vi "VILab.vi"() -> ()   [LabVIEW 2026, in "VILab.lvlib"]
uses:
  VILab.lvlib
  CTLs/VILab State Data.ctl
  Classes/Tree Manager/Tree Manager.lvclass
  CTLs/Resource.ctl
  Classes/Data Item/Data Item.lvclass
  <vilib>/Utility/error.llb/Clear Errors.vi
  SubVIs/Decompose VI (Refnum).vi
  SubVIs/FaKI State Machine/FaKI State Machine.lvlib
panel:
  in  "Dissect":bool
  in  "Rebuild":bool
  in  "Properties":bool
  in  "Clone":bool
  in  "Delete":bool
  in  "Add":bool
  in  "Tree":string(tree)
  # "WARNING:\nThis unofficial utility has NO WARRANTY and uses internal LabVIEW functionality that is NOT supported by National Instruments.\nYou will very likely crash LabVIEW and create insane/corrupted VI's, so use this at your own risk. But that's all part of the Fun™, right? ;)"
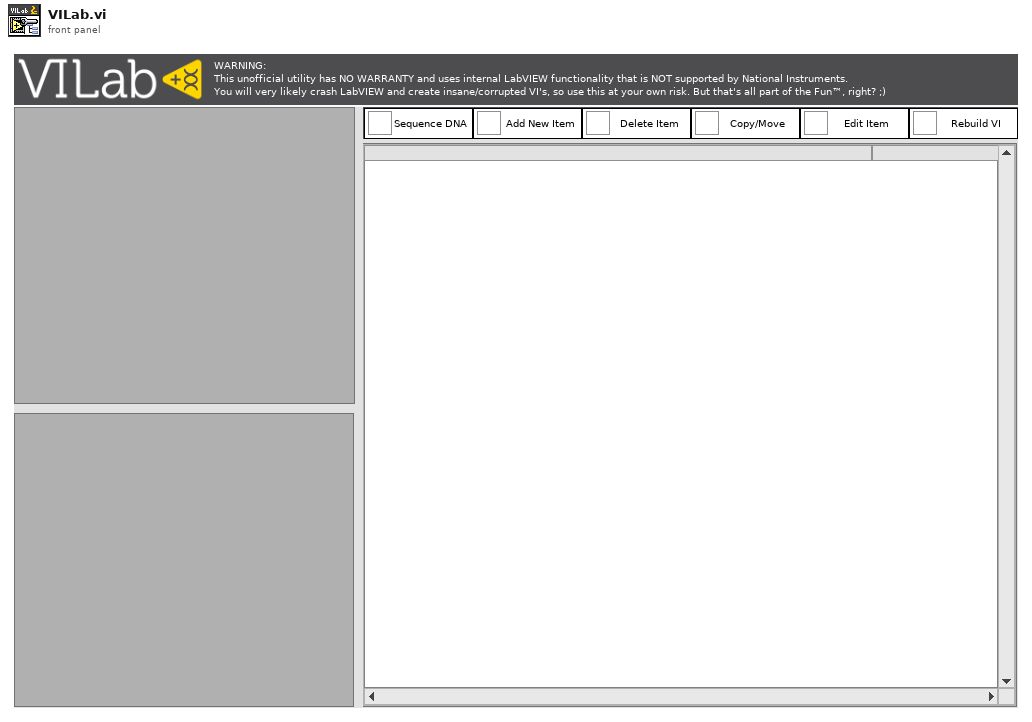
[diagram p1: front panel]
types:
  T1 = typedef "VILab.lvlib/VILab State Data.ctl" = cluster{"Core":cluster{"Current VI Reference":refnum<vi>, "Close Panel on Exit?":bool}, "Embedded VI":refnum<vi>, "Def VI Res":T2[], "Tree Mgr":refnum<class "Tree Manager.lvclass">, "Data":refnum<class "Data Item.lvclass">[]}
  T2 = typedef "VILab.lvlib/Resource.ctl" = cluster{"type":u32, "id":i32, "name":string, "binary data":string}
  T3 = enum32{"Invalid", "Standard", "Closed", "Hidden", "Minimized", "Maximized"}
  T4 = enum32{"invalid app kind", "Development System", "Run Time System", "Student Edition", "Embedded LabVIEW", "Evaluation", "Custom"}
  T5 = cluster{"Current VI Reference":refnum<vi>, "Close Panel on Exit?":bool}
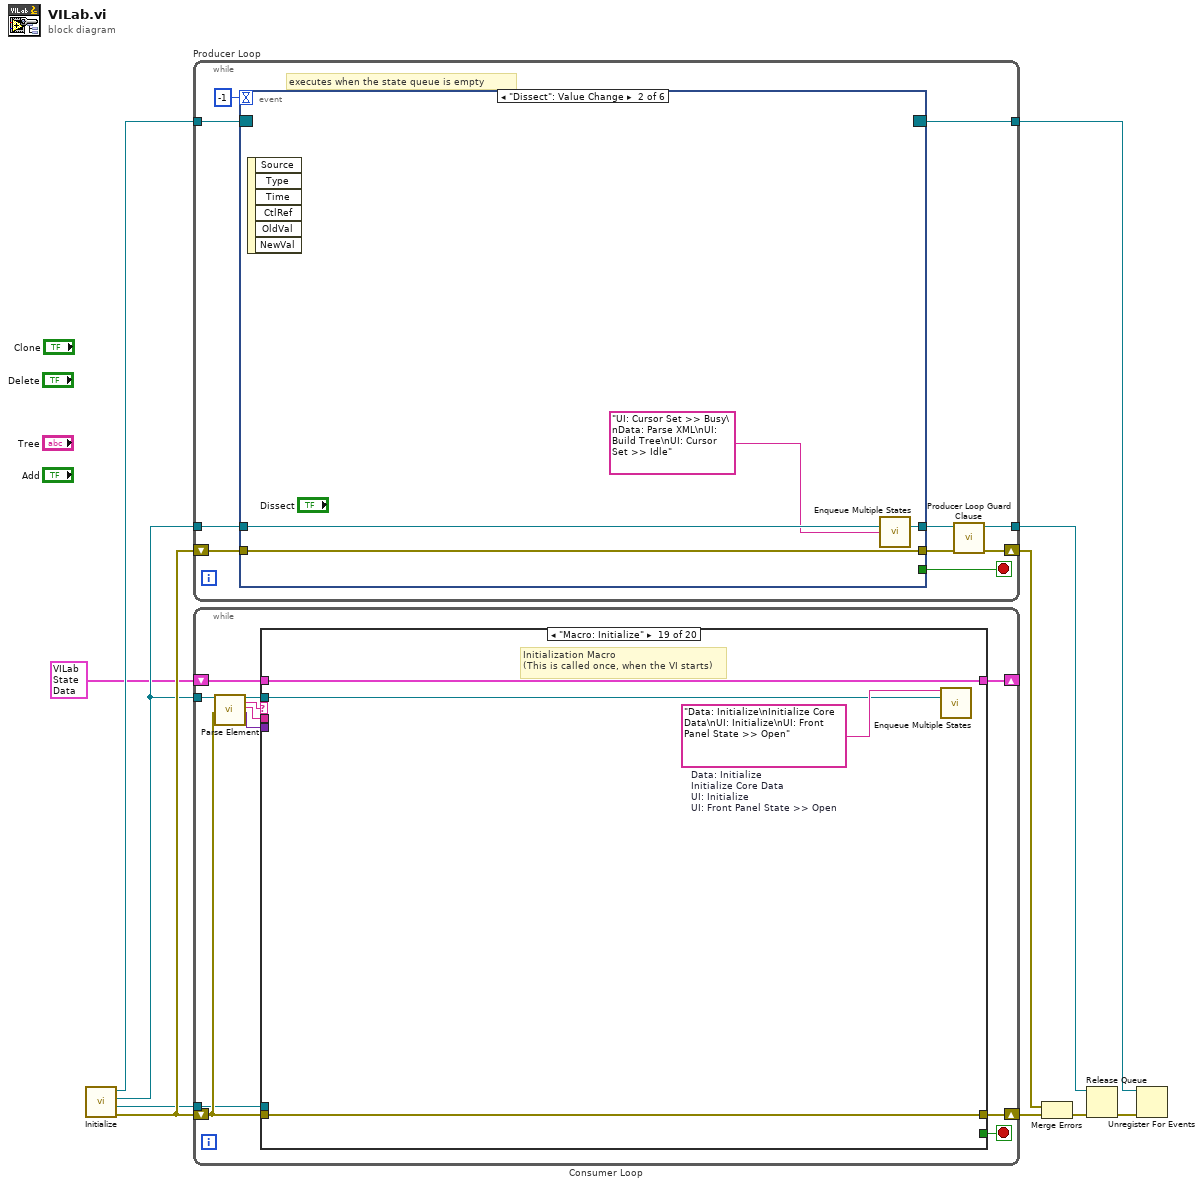
[diagram p0: block diagram]
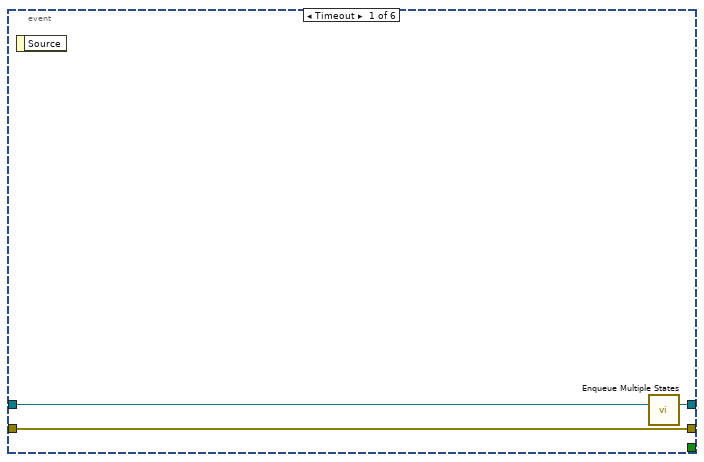
[diagram p2: hidden frame]
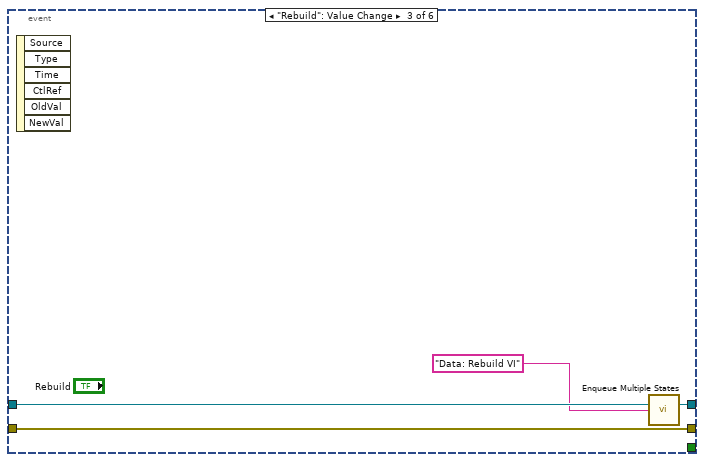
[diagram p3: hidden frame]
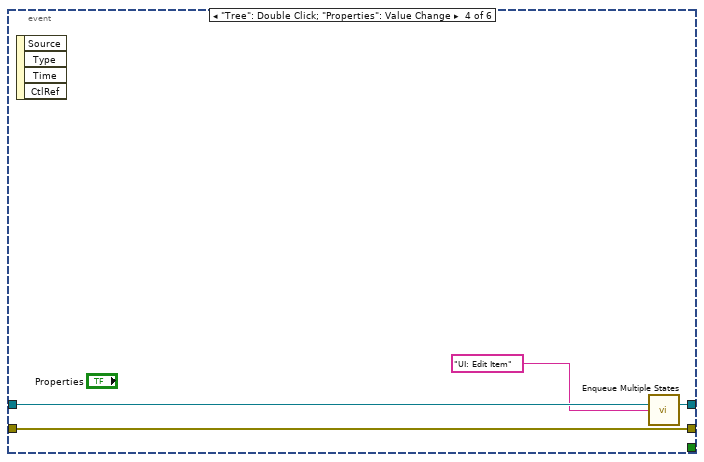
[diagram p4: hidden frame]
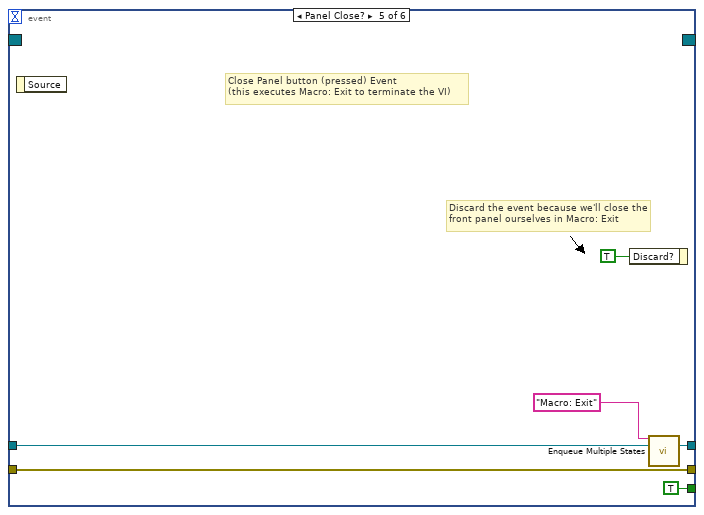
[diagram p5: hidden frame]
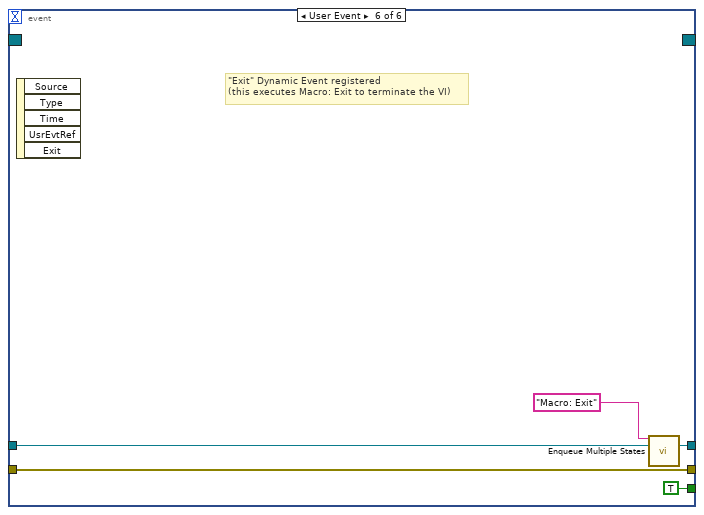
[diagram p6: hidden frame]
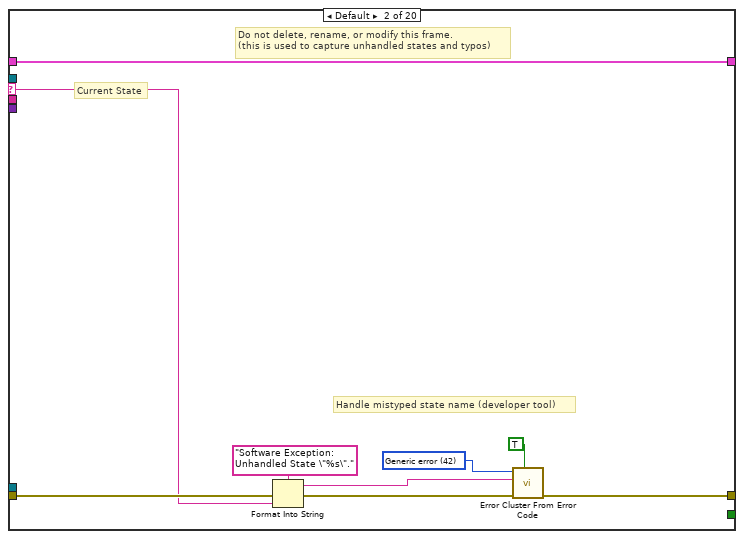
[diagram p8: hidden frame]
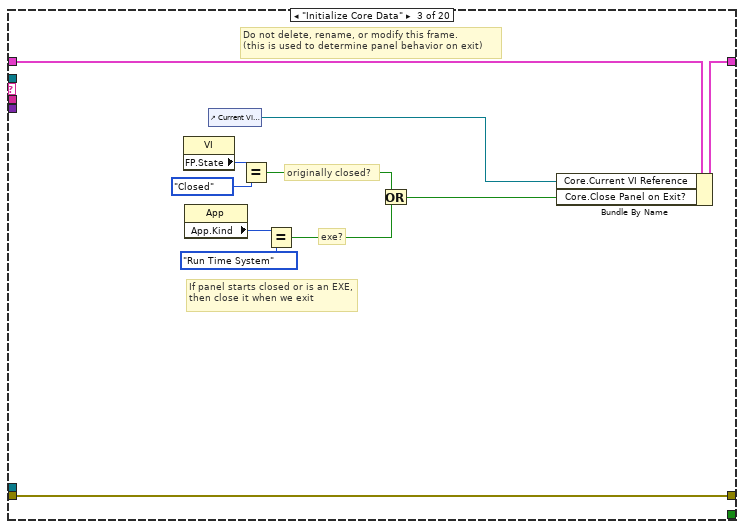
[diagram p9: hidden frame]
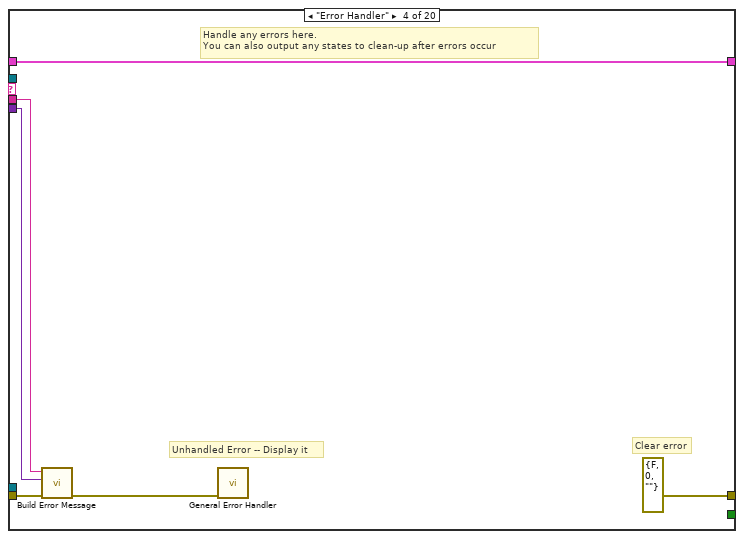
[diagram p10: hidden frame]
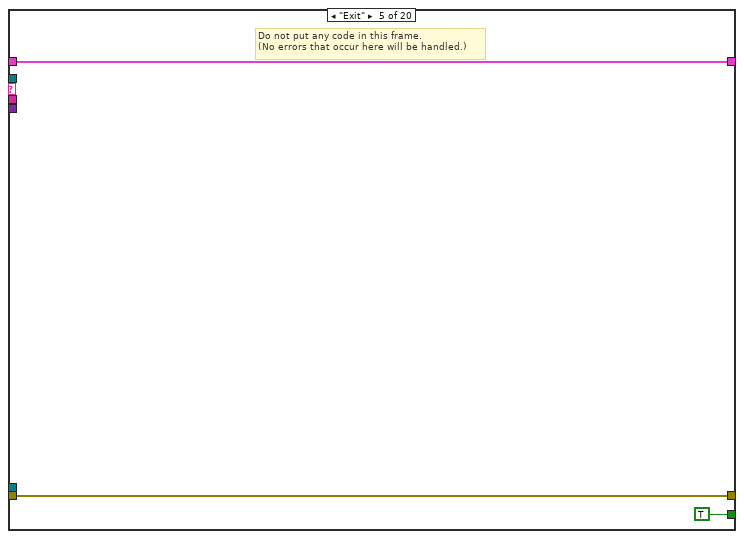
[diagram p11: hidden frame]
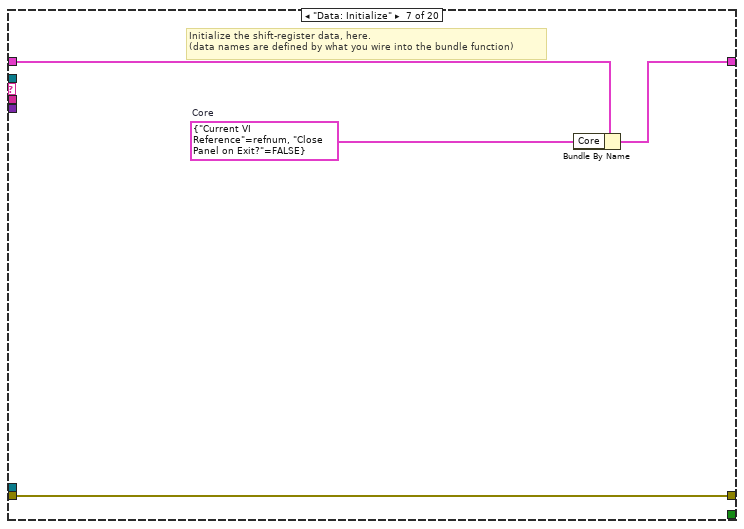
[diagram p13: hidden frame]
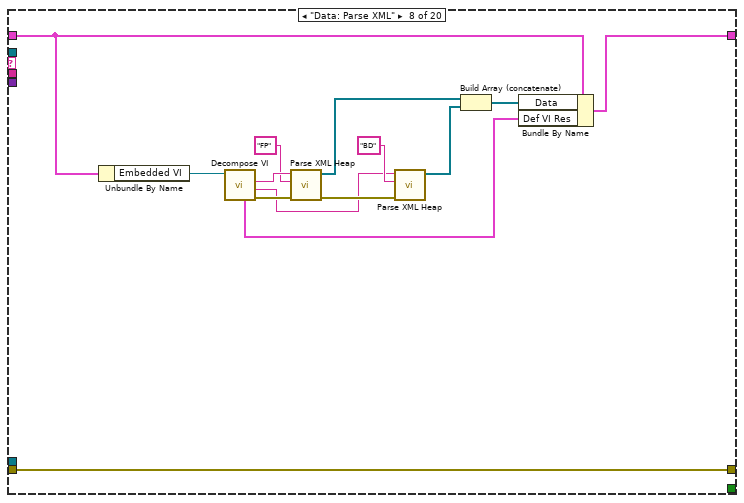
[diagram p14: hidden frame]
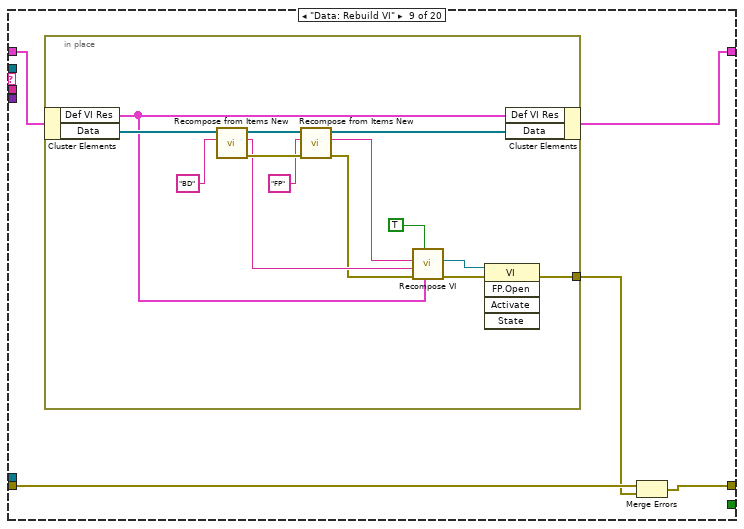
[diagram p15: hidden frame]
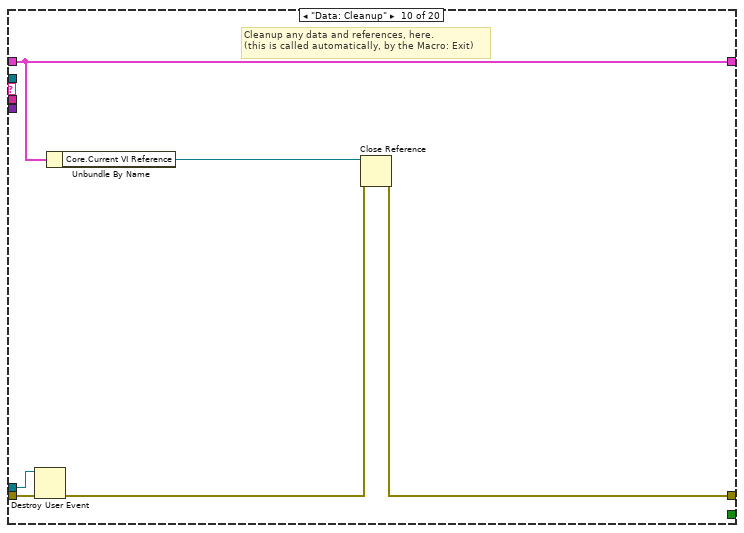
[diagram p16: hidden frame]
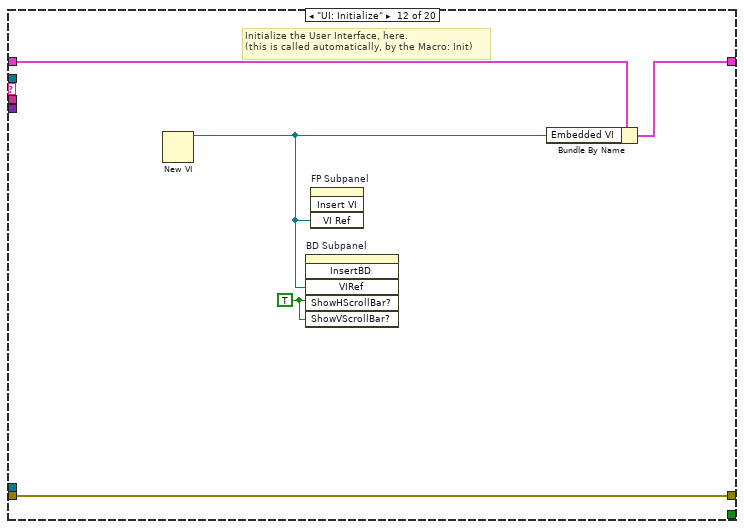
[diagram p18: hidden frame]
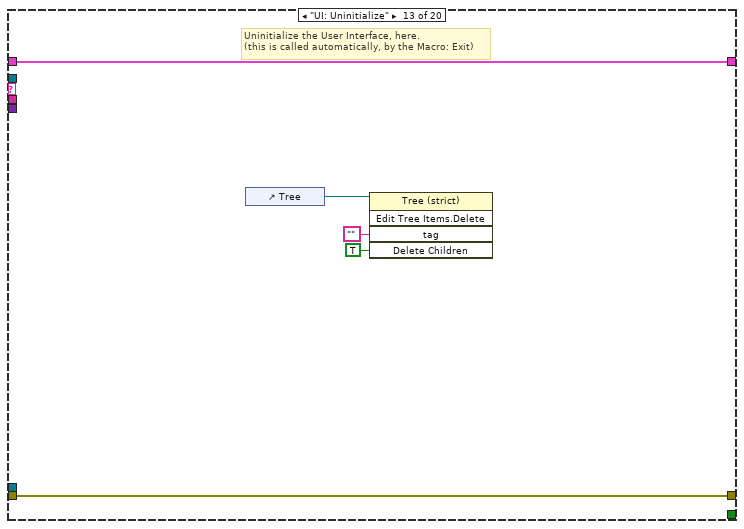
[diagram p19: hidden frame]
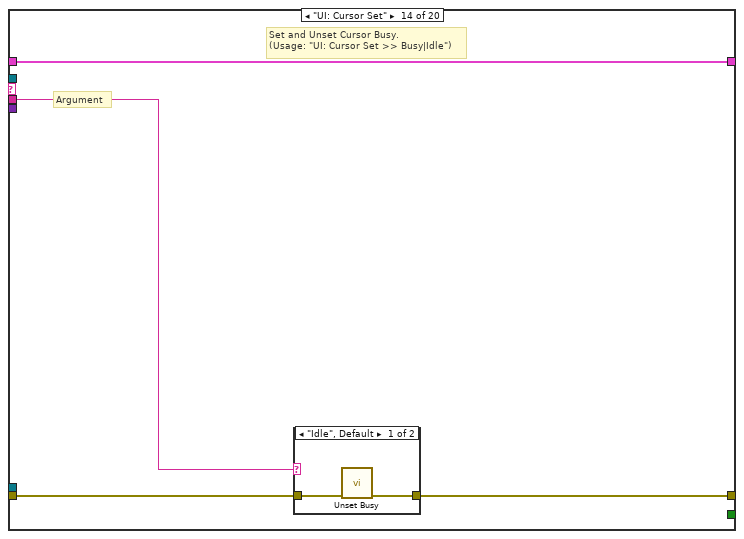
[diagram p20: hidden frame]
diagram:
  n1 = call "Initialize.vi"() -> ("error out"=w7:errorcluster, "Exit Event out"=w4:refnum<user-event>, "queue out"=w6:refnum<queue>, "Event Registration Refnum out"=w5:refnum<event-registration>)  [unwired: 8 in]
  n2 = while "Producer Loop" {
    shift-right: [w16] -> w10
    shift-left: w7 -> [w21]
    tunnel: w5 -> [w13]
    tunnel: w6 -> [w19]
    tunnel: [w14] -> w8
    tunnel: [w12] -> w2
    stop <- w18 stop-if-true
    # "executes when the state queue is empty"
    n3 = event shown="[1] \"Dissect\": Value Change" {
      selector: w13 -> [_ _ _ _ _ _]
      dyn-events: [_ _ _ _ _ _] -> w12
      timeout: -1 ("Timeout") -> [_ _ _ _ _ _]
      tunnel: [w22 w26 w30 w34 w42 w47] -> w17
      tunnel: w21 -> [w22 w26 w30 w34 w42 w47]
      tunnel: w19 -> [w23 w27 w31 w35 w39 w45]
      tunnel: [w24 w28 w32 w36 w38 w44] -> w15
      tunnel: [_ _ _ _ TRUE TRUE] -> w18
      event Timeout {
        n4 = event-data() -> ()  [unwired: 1 in, 1 out]
        n5 = call "Enqueue Multiple States.vi"("queue in"=w23) -> ("queue out"=w24:refnum<queue>)  [unwired: 14 in]
      }
      event "Dissect": Value Change {
        n6 = event-data() -> ()  [unwired: 1 in, 6 out]
        n7 = call "Enqueue Multiple States.vi"("queue in"=w27, "State(s) at Back"="UI: Cursor Set >> Busy\nData: Parse XML\nUI: Build Tree\nUI: Cursor Set >> Idle") -> ("queue out"=w28:refnum<queue>)  [unwired: 13 in]
      }
      event "Rebuild": Value Change {
        n8 = event-data() -> ()  [unwired: 1 in, 6 out]
        n9 = call "Enqueue Multiple States.vi"("queue in"=w31, "State(s) at Back"="Data: Rebuild VI") -> ("queue out"=w32:refnum<queue>)  [unwired: 13 in]
      }
      event "Tree": Double Click; "Properties": Value Change {
        n10 = event-data() -> ()  [unwired: 1 in, 4 out]
        n11 = call "Enqueue Multiple States.vi"("queue in"=w35, "State(s) at Back"="UI: Edit Item") -> ("queue out"=w36:refnum<queue>)  [unwired: 13 in]
      }
      event Panel Close? {
        # "Discard the event because we'll close the front panel ourselves in Macro: Exit"
        # "Close Panel button (pressed) Event\n(this executes Macro: Exit to terminate the VI)"
        n12 = event-data() -> ()  [unwired: 1 in, 1 out]
        n13 = event-data("Discard?"=TRUE) -> ()  [unwired: 1 in, 1 out]
        n14 = call "Enqueue Multiple States.vi"("State(s) at Front"="Macro: Exit", "queue in"=w39) -> ("queue out"=w38:refnum<queue>)  [unwired: 13 in]
      }
      event User Event {
        # "\"Exit\" Dynamic Event registered\n(this executes Macro: Exit to terminate the VI)"
        n15 = event-data() -> ()  [unwired: 1 in, 5 out]
        n16 = call "Enqueue Multiple States.vi"("State(s) at Front"="Macro: Exit", "queue in"=w45) -> ("queue out"=w44:refnum<queue>)  [unwired: 13 in]
      }
    }
    n17 = call "Producer Loop Guard Clause.vi"("error in (no error)"=w17, "queue in"=w15) -> ("error out"=w16:errorcluster, "queue out"=w14:refnum<queue>)  [unwired: 8 in]
  }
  n18 = while "Consumer Loop" {
    shift-right: [w55] -> _
    shift-left: T1 {"Core"={"Current VI Reference"=refnum, "Close Panel on Exit?"=FALSE}, "Embedded VI"=refnum, "Def VI Res"=[], "Tree Mgr"=refnum, "Data"=[]} ("Resource Editor State Data") -> [w54]
    shift-right: [w58] -> w11
    shift-left: w7 -> [w57]
    tunnel: w6 -> [w53]
    tunnel: w4 -> [w48]
    stop <- w56 stop-if-true
    n19 = call "Parse Element.vi"("queue in"=w53, "error in (no error)"=w57) -> ("queue out"=w52:refnum<queue>, "State"=w51:string, "Arg"=w50:string, "Data"=w49:variant)  [unwired: 14 in]
    n20 = case shown="\"Macro: Initialize\"" w51 {
      selector: w51 -> [_ w61 _ _ _ _ _ _ _ _ _ _ _ _ _ _ _ _ _ _]
      tunnel: w52 -> [_ _ _ _ _ _ _ _ _ _ _ _ _ _ _ w226 _ _ w269 w277]
      tunnel: w50 -> [_ _ _ w81 _ _ _ _ _ _ _ _ _ w147 w155 _ _ _ _ _]
      tunnel: w54 -> [w59 w63 w75 w85 w88 w90 w94 w107 w112 w132 w135 w140 w145 w148 w157 w229 w252 w267 w271 w281]
      tunnel: [w60 w68 w80 errorcluster {"status"=FALSE, "code"=0, "source"=""} ("error out") w89 w91 w95 w109 w111 w134 w136 w141 w146 w149 w158 w227 w249 w268 w272 w282] -> w58
      tunnel: w57 -> [w60 w67 w80 w84 w89 w91 w95 w109 w114 w131 w136 w141 w146 w150 w159 w227 w250 w268 w272 w282]
      tunnel: [_ _ _ _ TRUE _ _ _ _ _ _ _ _ _ _ _ _ _ _ _] -> w56
      tunnel: [w59 w63 w79 w85 w88 w90 w92 w108 w113 w132 w135 w139 w145 w148 w157 w228 w251 w267 w271 w281] -> w55
      tunnel: w49 -> [_ _ _ w82 _ _ _ _ _ _ _ _ _ _ _ _ _ _ _ _]
      tunnel: w48 -> [_ _ _ _ _ _ _ _ _ w130 _ _ _ _ _ _ _ _ _ _]
      frame "---------- Core ----------" {
        # "Do not put any code in this frame.\n(it is a separator no-op)"
      }
      frame Default {
        w65 = 42 items=["No error", "Argument error", "Memory is full", "Out of zone", "End of file", "File already open", "Generic file I/O error", "File not found", "File permission error", "Disk is full", "Duplicate path", "Too many files open", "System feature not enabled", "Resource file not found", "Cannot add resource", "Resource not found", "Image not found", "Image memory error", "Pen does not exist", "Config type invalid", "Config token not found", "Config parse error", "Config memory error", "Bad external code format", "Bad external code offset", "External code not present", "Null window", "Destroy window error", "Null menu", "Print aborted", "Bad print record", "Print driver error", "Windows error during printing", "Memory error during printing", "Print dialog error", "Generic print error", "Invalid device refnum", "Device not found", "Device parameter error", "Device unit error", "Cannot open device", "Device call aborted", "Generic error", "Cancelled by user", "Object ID too low", "Object ID too high", "Object not in heap", "Unknown heap", "Unknown object (invalid DefProc)", "Unknown object (DefProc not in table)", "Message out of range", "Invalid (null) method", "Unknown message", "Manager call not supported", "Bad address", "Network operation in progress", "Network operation timed out", "Connection is busy", "Network attribute not supported", "Network error", "Address in use", "System out of memory", "Connection aborted", "Connection refused", "Not connected", "Already connected", "Connection closed", "Initialization error (interapplication manager)", "Bad occurrence", "Wait on unbound occurrence handler", "Occurrence queue overflow", "Datalog type conflict", "Unused", "Unrecognized type (interapplication manager)", "Memory corrupt", "Failed to make temporary DLL", "Old CIN version", "Drag socket not found", "Failed to load drop-object", "Failed to register OLE object", "Failed to release OLE object", "Format specifier type mismatch", "Unknown format specifier", "Too few format specifiers", "Too many format specifiers", "Scan failed", "Newer CIN version", "Error converting to variant", "Runtime menu error", "Password tampered", "Variant attribute not found", "Incompatible variant data type", "Event data is not available", "Event Store is not present", "Occurrence is not found", "Event Queue is not created", "Event info is not available", "Refnum passed is NULL", "Error retrieving Class GUID", "Error retrieving CoClass GUID", "Error retrieving TypeLib GUID.", "Bad built application magic bytes.", "Specific driver is different from the specific driver associated with the Logical Name.", "There is no session opened to the class driver.", "Max Error", "MAX - Error with config objects", "MAX - Error loading configuration", "MAX - Group not supported"]
        # "Current State"
        # "Do not delete, rename, or modify this frame.\n(this is used to capture unhandled states and typos)"
        # "Handle mistyped state name (developer tool)"
        n21 = Format Into String(format string="Software Exception: Unhandled State \"%s\"." ("message"), error in=w67, w61) -> (resulting string=w64:string, error out=w69:errorcluster)  [unwired: 1 in]
        n22 = call <vilib>:"Error Cluster From Error Code.vi"("show call chain? (False)"=TRUE, "error in (no error)"=w69, "error message (\"\")"=w64, "error code (0)"=w65) -> ("error out"=w68:errorcluster)  [unwired: 5 in]
      }
      frame "Initialize Core Data" {
        # "Do not delete, rename, or modify this frame.\n(this is used to determine panel behavior on exit)"
        # "originally closed?"
        # "exe?"
        # "If panel starts closed or is an EXE, then close it when we exit"
        n23 = property class="VI"() -> ("FP.State"=w72:T3)  [unwired: 2 in, 2 out]
        n24 = property class="App"() -> ("App.Kind"=w78:T4)  [unwired: 2 in, 2 out]
        n25 = control-ref of="Current VI Reference"() -> (w73:refnum<vi>)
        n26 = Equal?(x=w72, y=T3."Closed" ("Front Panel Window:State")) -> (x = y?=w70:bool)
        n27 = Equal?(x=w78, y=T4."Run Time System" ("Application:Kind")) -> (x = y?=w76:bool)
        n28 = Or(x=w70, y=w76) -> (x .or. y?=w74:bool)
        n29 = Bundle By Name(cluster=w75, "Core.Current VI Reference"=w73, "Core.Close Panel on Exit?"=w74) -> (w79:T1)
      }
      frame "Error Handler" {
        # "Unhandled Error -- Display it"
        # "Handle any errors here.\nYou can also output any states to clean-up after errors occur"
        # "Clear error"
        n30 = call "Build Error Message.vi"("error in (no error)"=w84, "Data"=w82, "Arg"=w81) -> ("error out"=w83:errorcluster)  [unwired: 8 in]
        n31 = call <vilib>:"General Error Handler.vi"("error in (no error)"=w83) -> ()  [unwired: 10 in, 5 out]
      }
      frame "Exit" {
        # "Do not put any code in this frame.\n(No errors that occur here will be handled.)"
      }
      frame "---------- Data ----------" {
        # "Do not put any code in this frame.\n(It is a separator no-op. You can make a copy of this frame to create a new Data frame)"
      }
      frame "Data: Initialize" {
        w93 = T5 {"Current VI Reference"=refnum, "Close Panel on Exit?"=FALSE}  # Core
        # "Initialize the shift-register data, here.\n(data names are defined by what you wire into the bundle function)"
        n32 = Bundle By Name(cluster=w94, "Core"=w93) -> (w92:T1)
      }
      frame "Data: Parse XML" {
        n33 = Unbundle By Name(w107) -> ("Embedded VI"=w106:refnum<vi>)
        n34 = call-poly "Decompose VI.vi"("VI Ref"=w106) -> ("error out"=w104:errorcluster, "Block Diagram XML"=w100:string, "Front Panel XML"=w105:string, "Other resources"=w96:T2[])  [unwired: 6 in, 1 out]
        n35 = call "Parse XML Heap.vi"("error in (no error)"=w104, "Root Parent"="FP", "XML"=w105) -> ("error out"=w101:errorcluster, "Items"=w99:refnum<class "Data Item.lvclass">[])  [unwired: 7 in]
        n36 = call "Parse XML Heap.vi"("error in (no error)"=w101, "Root Parent"="BD", "XML"=w100) -> ("Items"=w98:refnum<class "Data Item.lvclass">[])  [unwired: 7 in, 1 out]
        n37 = Build Array (concatenate)(w99, w98) -> (w97:refnum<class "Data Item.lvclass">[])
        n38 = Bundle By Name(cluster=w107, "Data"=w97, "Def VI Res"=w96) -> (w108:T1)
      }
      frame "Data: Rebuild VI" {
        n39 = in-place {
          in-place-border: [w119] -> w110
          n40 = in-place-cluster #1(w112) -> ("Def VI Res"=w116:T2[], "Data"=w122:refnum<class "Data Item.lvclass">[])
          n41 = call "Recompose from Items New.vi"("Tree Tag"="BD", "All Data"=w122) -> ("error out"=w128:errorcluster, "XML String"=w126:string, "All Data out"=w115:refnum<class "Data Item.lvclass">[])  [unwired: 7 in]
          n42 = call "Recompose from Items New.vi"("error in (no error)"=w128, "Tree Tag"="FP", "All Data"=w115) -> ("error out"=w120:errorcluster, "XML String"=w127:string, "All Data out"=w121:refnum<class "Data Item.lvclass">[])  [unwired: 6 in]
          n43 = call "Recompose VI.vi"("Other resources (default)"=w116, "Open VI? (F)"=TRUE, "error in (no error)"=w120, "Block Diagram XML"=w126, "Front Panel XML"=w127) -> ("error out"=w124:errorcluster, "VI Refnum (if opened)"=w123:refnum<vi>)  [unwired: 4 in, 1 out]
          n44 = invoke class="VI" method="FP.Open"(reference=w123, error in=w124) -> (error out=w119:errorcluster)  [unwired: 3 in, 4 out]
          n45 = in-place-cluster #1("Def VI Res"=w116, "Data"=w121) -> (w113:T1)
        }
        n46 = Merge Errors(w114, w110) -> (w111:errorcluster)
      }
      frame "Data: Cleanup" {
        # "Cleanup any data and references, here.\n(this is called automatically, by the Macro: Exit)"
        n47 = Destroy User Event(user event=w130, error in=w131) -> (error out=w129:errorcluster)
        n48 = Unbundle By Name(w132) -> ("Core.Current VI Reference"=w133:refnum<vi>)
        n49 = Close Reference(reference=w133, error in (no error)=w129) -> (error out=w134:errorcluster)
      }
      frame "---------- UI ----------" {
        # "Do not put any code in this frame.\n(It is a separator no-op. You can make a copy of this frame to create a new UI frame)"
      }
      frame "UI: Initialize" {
        w138 = TRUE ("ShowHScrollBar")
        # "Initialize the User Interface, here.\n(this is called automatically, by the Macro: Init)"
        n50 = New VI() -> (3:w137:refnum<vi>)  [unwired: 7 in, 1 out]
        n51 = invoke on="BD Subpanel" class="SubPnl" method="InsertBD"("VIRef"=w137, "ShowHScrollBar?"=w138, "ShowVScrollBar?"=w138) -> ()  [unwired: 3 in, 6 out]
        n52 = invoke on="FP Subpanel" class="SubPnl" method="Insert VI"("VI Ref"=w137) -> ()  [unwired: 3 in, 4 out]
        n53 = Bundle By Name(cluster=w140, "Embedded VI"=w137) -> (w139:T1)
      }
      frame "UI: Uninitialize" {
        # "Uninitialize the User Interface, here.\n(this is called automatically, by the Macro: Exit)"
        n54 = control-ref of="Tree"() -> (w144:refnum<vi>)
        n55 = invoke class="Tree (strict)" method="Edit Tree Items.Delete"(reference=w144, "tag"="", "Delete Children"=TRUE ("Delete Children?")) -> ()  [unwired: 2 in, 5 out]
      }
      frame "UI: Cursor Set" {
        # "Argument"
        # "Set and Unset Cursor Busy.\n(Usage: \"UI: Cursor Set >> Busy|Idle\")"
        n56 = case shown="\"Idle\", Default" w147 {
          tunnel: w150 -> [w152 w154]
          tunnel: [w151 w153] -> w149
          frame "Idle", Default {
            n57 = call <vilib>:"Unset Busy.vi"("error in (no error)"=w152) -> ("error out"=w151:errorcluster)  [unwired: 10 in]
          }
          frame "Busy" {
            n58 = call <vilib>:"Set Busy.vi"("error in (no error)"=w154) -> ("error out"=w153:errorcluster)  [unwired: 9 in, 1 out]
          }
        }
      }
      frame "UI: Front Panel State" {
        # "Argument"
        # "Set Front Panel Open or Closed\n(Usage: \"UI: Front Panel State >> Open|Close\")"
        n59 = Unbundle By Name(w157) -> ("Core.Current VI Reference"=w156:refnum<vi>)
        n60 = case shown="\"Open\", \"Standard\", Default" w155 {
          tunnel: w159 -> [w166 w180 w192 w205 w218]
          tunnel: [w167 w181 w193 w206 w219] -> w158
          tunnel: w156 -> [w164 w178 w190 w203 w216]
          frame "Open", "Standard", Default {
            w160 = T3."Standard" ("State")
            n61 = property class="VI"(reference=w164, error in=w166) -> (reference out=w163:refnum<vi>, error out=w165:errorcluster, "FP.State"=w162:T3)
            n62 = Not Equal?(x=w162, y=w160) -> (x != y?=w161:bool)
            n63 = case shown="True" w161 {
              tunnel: [w172 w173] -> w167
              tunnel: w165 -> [w171 w173]
              tunnel: w163 -> [w169 _]
              tunnel: w160 -> [w168 _]
              frame True {
                n64 = invoke class="VI" method="FP.Open"(reference=w169, error in=w171, "Activate"=TRUE, "State"=w168) -> (error out=w172:errorcluster)  [unwired: 1 in, 4 out]
              }
              frame False {
              }
            }
          }
          frame "Close", "Closed" {
            n65 = property class="VI"(reference=w178, error in=w180) -> (reference out=w177:refnum<vi>, error out=w179:errorcluster, "FP.State"=w175:T3)
            n66 = Not Equal?(x=w175, y=T3."Closed" ("Front Panel Window:State")) -> (x != y?=w174:bool)
            n67 = case shown="True" w174 {
              tunnel: [w182 w185] -> w181
              tunnel: w179 -> [w182 w184]
              tunnel: w177 -> [_ w183]
              frame False {
              }
              frame True {
                n68 = invoke class="VI" method="FP.Close"(reference=w183, error in=w184) -> (error out=w185:errorcluster)  [unwired: 1 in, 2 out]
              }
            }
          }
          frame "Hidden", "Hide" {
            w186 = T3."Hidden" ("State")
            n69 = property class="VI"(reference=w190, error in=w192) -> (reference out=w189:refnum<vi>, error out=w191:errorcluster, "FP.State"=w188:T3)
            n70 = Not Equal?(x=w188, y=w186) -> (x != y?=w187:bool)
            n71 = case shown="True" w187 {
              tunnel: [w197 w198] -> w193
              tunnel: w191 -> [w196 w198]
              tunnel: w189 -> [w195 _]
              tunnel: w186 -> [w194 _]
              frame True {
                n72 = invoke class="VI" method="FP.Open"(reference=w195, error in=w196, "State"=w194) -> (error out=w197:errorcluster)  [unwired: 2 in, 4 out]
              }
              frame False {
              }
            }
          }
          frame "Minimize", "Minimized" {
            w199 = T3."Minimized" ("State")
            n73 = property class="VI"(reference=w203, error in=w205) -> (reference out=w202:refnum<vi>, error out=w204:errorcluster, "FP.State"=w201:T3)
            n74 = Not Equal?(x=w201, y=w199) -> (x != y?=w200:bool)
            n75 = case shown="True" w200 {
              tunnel: [w210 w211] -> w206
              tunnel: w204 -> [w209 w211]
              tunnel: w202 -> [w208 _]
              tunnel: w199 -> [w207 _]
              frame True {
                n76 = invoke class="VI" method="FP.Open"(reference=w208, error in=w209, "State"=w207) -> (error out=w210:errorcluster)  [unwired: 2 in, 4 out]
              }
              frame False {
              }
            }
          }
          frame "Maximize", "Maximized" {
            w212 = T3."Maximized" ("State")
            n77 = property class="VI"(reference=w216, error in=w218) -> (reference out=w215:refnum<vi>, error out=w217:errorcluster, "FP.State"=w214:T3)
            n78 = Not Equal?(x=w214, y=w212) -> (x != y?=w213:bool)
            n79 = case shown="True" w213 {
              tunnel: [w223 w224] -> w219
              tunnel: w217 -> [w222 w224]
              tunnel: w215 -> [w221 _]
              tunnel: w212 -> [w220 _]
              frame True {
                n80 = invoke class="VI" method="FP.Open"(reference=w221, error in=w222, "State"=w220) -> (error out=w223:errorcluster)  [unwired: 2 in, 4 out]
              }
              frame False {
              }
            }
          }
        }
      }
      frame "UI: Edit Item" {
        n81 = in-place {
          in-place-border: [w230] -> w225
          n82 = in-place-cluster #2(w229) -> ("Data"=w236:refnum<class "Data Item.lvclass">[])
          n83 = local read "Tree"() -> (w240:string)
          n84 = call "Find Item by Tag.vi"("Tree Tag"=w240, "All Data"=w236) -> ("Index"=w238:i32, "All Data out"=w239:refnum<class "Data Item.lvclass">[])  [unwired: 7 in, 1 out]
          n85 = in-place {
            in-place-border: [w247] -> w237
            in-place-border: [w246] -> w231
            in-place-border: w236 -> [w245]
            n86 = in-place-array #3(w239, w238) -> (w248:refnum<class "Data Item.lvclass">)
            n87 = call-dynamic "Edit Data.vi"("All Data"=w245, "Data Item in"=w248) -> ("OK?"=w246:bool, "Data Item out"=w247:refnum<class "Data Item.lvclass">)  [unwired: 6 in, 2 out]
            n88 = in-place-array #3(w247) -> (w235:refnum<class "Data Item.lvclass">[])  [unwired: 1 out]
          }
          n89 = case shown="True" w231 {
            tunnel: w235 -> [w241 w242]
            tunnel: [w241 w243] -> w234
            tunnel: w237 -> [_ w244]
            frame False {
            }
            frame True {
              n90 = call-dynamic "Update Item.vi"("All Data"=w242, "Data Item in"=w244) -> ("All Data out"=w243:refnum<class "Data Item.lvclass">[])  [unwired: 7 in, 2 out]
            }
          }
          n91 = Select(t="UI: Build Tree", s=w231, f="") -> (s? t:f=w230:string)
          n92 = in-place-cluster #2("Data"=w234) -> (w228:T1)
        }
        n93 = call "Enqueue Multiple States.vi"("queue in"=w226, "State(s) at Back"=w225) -> ()  [unwired: 13 in, 1 out]
      }
      frame "UI: Build Tree" {
        n94 = in-place {
          in-place-border: w250 -> [w253]
          in-place-border: [w259] -> w249
          n95 = in-place-cluster #4(w252) -> ("Data"=w260:refnum<class "Data Item.lvclass">[])  [unwired: 1 out]
          n96 = control-ref of="Tree"() -> (w256:refnum<vi>)
          n97 = call "Init Tree Control.vi"("error in (no error)"=w253, "TreeControl in"=w256) -> ("error out"=w257:errorcluster, "TreeControl out"=w258:refnum<vi>)  [unwired: 8 in]
          n98 = call "Create Tree Manager.vi"("error in (no error)"=w257, "Tree Control"=w258) -> ("error out"=w255:errorcluster, "Tree Manager"=w254:refnum<class "Tree Manager.lvclass">)  [unwired: 8 in]
          n99 = for {
            shift-right: [w265] -> w261
            shift-left: w254 -> [w266]
            tunnel: w260 -> [w264] mode=indexing
            shift-right: [w262] -> w259
            shift-left: w255 -> [w263]
            n100 = call "Add Item to Tree.vi"("error in (no error)"=w263, "Data Item"=w264, "Tree Manager in"=w266) -> ("error out"=w262:errorcluster, "Tree Manager out"=w265:refnum<class "Tree Manager.lvclass">)  [unwired: 6 in, 1 out]
          }
          n101 = in-place-cluster #4("Data"=w260, "Tree Mgr"=w261) -> (w251:T1)
        }
      }
      frame "---------- Macro ----------" {
        # "Do not put any code in this frame.\n(It is a separator no-op. You can make a copy of this frame to create a new Macro frame)"
      }
      frame "Macro: Initialize" {
        w270 = "Data: Initialize\nInitialize Core Data\nUI: Initialize\nUI: Front Panel State >> Open"  # Data: Initialize Initialize Core Data UI: Initialize UI: Front Panel State >> Open
        # "Initialization Macro\n(This is called once, when the VI starts)"
        n102 = call "Enqueue Multiple States.vi"("State(s) at Front"=w270, "queue in"=w269) -> ()  [unwired: 13 in, 1 out]
      }
      frame "Macro: Exit" {
        # "Exit Macro\n(This is called once, when the VI exits)"
        n103 = Unbundle By Name(w281) -> ("Core.Close Panel on Exit?"=w280:bool)
        n104 = Select(t="UI: Front Panel State >> Close\n", s=w280, f="") -> (s? t:f=w276:string)
        n105 = Concatenate Strings("UI: Uninitialize\n", w276, "Data: Cleanup\nExit") -> (w274:string)
        n106 = call "Enqueue Multiple States.vi"("State(s) at Front"=w274, "queue in"=w277) -> ()  [unwired: 13 in, 1 out]
      }
    }
  }
  n107 = Merge Errors(w10, w11) -> (w9:errorcluster)
  n108 = Release Queue(queue=w8, error in (no error)=w9) -> (error out=w3:errorcluster)  [unwired: 1 in, 2 out]
  n109 = Unregister For Events(event registration refnum=w2, error in=w3) -> ()  [unwired: 1 out]
